vi "Get Target to Host DMAMap.vi"(8 "error in (no error)":errorcluster, 11 "Item Ref in":T6 format="%.0x") -> (0 "error out":errorcluster, 2 "DMA configuration array":T1[](array[typedef]) {"reservation info"."reserver ref in" format="%.0x"}, 3 "Item Ref out":T6 format="%.0x")   [LabVIEW 2016]
uses:
  <vilib>/NI Veristand/Custom Device API/Custom Device Item Ref.ctl
  SubVIs/DMA Reservation.ctl
  <vilib>/rvi/FIFO/Fifo_Types/Fifo_DMA_Config.ctl
  <vilib>/rvi/DataTransferAndStorage/Container/Common/niFpgaDataTypeControl.ctl
  <vilib>/rvi/ClientSDK/Core/ModuleGeneration/CommunicationInterfaceUtility/niFpgaDmaChannelImplementation.ctl
  SubVIs/reservation info.ctl
  SubVIs/Channel Type.ctl
  <vilib>/NI Veristand/Custom Device API/Get Item Property (Variant).vi
  <vilib>/NI VeriStand/Custom Device API/Custom Device API.lvlib
  FPGA Addon System Explorer.lvlib
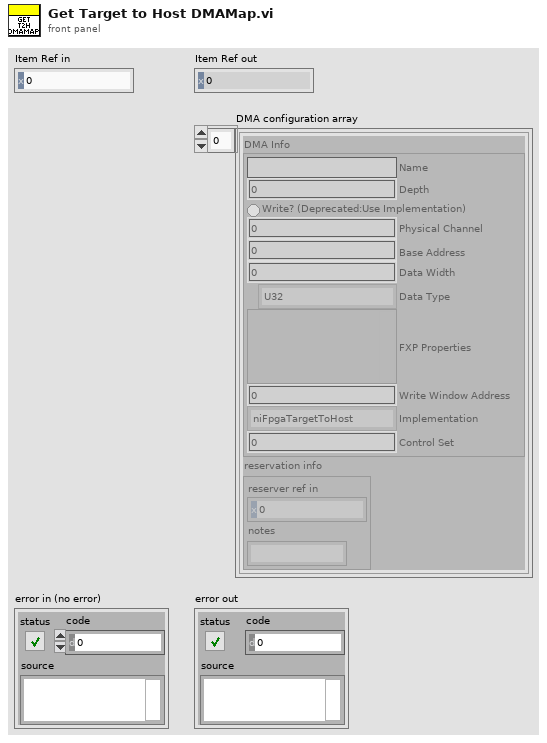
[diagram p1: front panel]
types:
  T1 = typedef "FPGA Addon System Explorer.lvlib/DMA Reservation.ctl" = cluster{"DMA Info":T2, "reservation info":T5}
  T2 = typedef "Fifo_DMA_Config.ctl" = cluster{"Name":string, "Depth":u32, "Write? (Deprecated:Use Implementation)":bool, "Physical Channel":u32, "Base Address":u32, "Data Width":u32, "Data Type":T3, "FXP Properties":variant, "Write Window Address":u32, "Implementation":T4, "Control Set":u32}
  T3 = typedef "niFpgaDataTypeControl.ctl" = enum32{"Boolean", "I8", "I16", "I32", "I64", "U8", "U16", "U32", "U64", "FXP", "CustomControl", "SGL"}
  T4 = typedef "niFpgaDmaChannelImplementation.ctl" = enum16{"niFpgaTargetToHost", "niFpgaHostToTarget", "niFpgaPeerToPeerWriter", "niFpgaPeerToPeerReader", "niCoreTargetToHost", "niCoreHostToTarget"}
  T5 = typedef "FPGA Addon System Explorer.lvlib/reservation info.ctl" = cluster{"reserver ref in":T6, "notes":string}
  T6 = typedef "Custom Device API.lvlib/Custom Device Item Ref.ctl" = u64
  T7 = typedef "FPGA Addon System Explorer.lvlib/Channel Type.ctl" = enum16{"Write Channel", "Read Channel", "Write Waveform", "Read Waveform"}
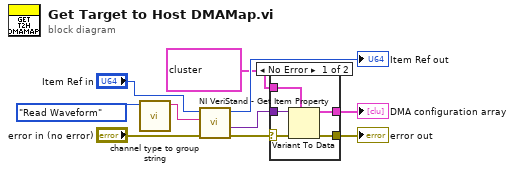
[diagram p0: block diagram]
diagram:
  n1 = call "channel type to group string.vi"("channel type"=Channel_Type."Read Waveform") -> ("FPGA.Controls"=w2:string)  [unwired: 10 in]
  n2 = call-poly <vilib>:"NI VeriStand - Get Item Property.vi"("error in (no error)"="error in (no error)", "Property Name"=w2, "Item Ref in"="Item Ref in") -> ("error out"=w6:errorcluster, "Value"=w7:variant, "Item Ref out"=→"Item Ref out":T6)  [unwired: 5 in, 1 out]
  n3 = case shown="No Error" w6 {
    selector: w6 -> [w13 w16]
    tunnel: [w15 w17] -> w3
    tunnel: w7 -> [w14 _]
    tunnel: [w12 w16] -> w5
    tunnel: T1[] [{"DMA Info"={"Name"="", "Depth"=0, "Write? (Deprecated:Use Implementation)"=FALSE, "Physical Channel"=0, "Base Address"=0, "Data Width"=0, "Data Type"=enum."U32", "FXP Properties"=variant, "Write Window Address"=0, "Implementation"=enum."niFpgaTargetToHost", "Control Set"=0}, "reservation info"={"reserver ref in"=0, "notes"=""}}, {"DMA Info"={"Name"="", "Depth"=0, "Write? (Deprecated:Use Implementation)"=FALSE, "Physical Channel"=0, "Base Address"=0, "Data Width"=0, "Data Type"=enum."U32", "FXP Properties"=variant, "Write Window Address"=0, "Implementation"=enum."niFpgaTargetToHost", "Control Set"=0}, "reservation info"={"reserver ref in"=0, "notes"=""}}] ("DMA configuration array") -> [w11 w17]
    frame No Error {
      n4 = Variant To Data(error in=w13, type=w11, Variant=w14) -> (data=w15:T1[], error out=w12:errorcluster)
    }
    frame Error {
    }
  }
  "error out" <- w5
  "DMA configuration array" <- w3
